vi "String To Anything.vi"(5 "Use Supplied":bool, 7 "Format String (%#_13g)":string="%#_13g", 8 "Error In":errorcluster, 9 "Strings":string[](array[string]), 10 "Type of Anything":variant, 11 "Read/Write Options":T1) -> (0 "Error Out":errorcluster, 3 "Variant":variant)   [LabVIEW 2020]
uses:
  SubVIs/Read Write Options Cluster.ctl
  SubVIs/Read Write Tag Lookup Cluster.ctl
  <vilib>/Utility/VariantDataType/Type.ctl
  <vilib>/Utility/VariantDataType/VariantType.lvlib
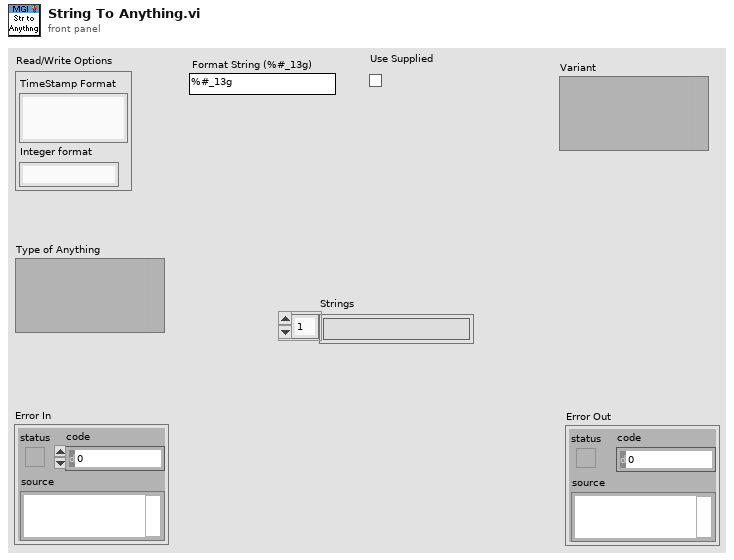
[diagram p1: front panel]
types:
  T1 = typedef "Read Write Options Cluster.ctl" = cluster{"TimeStamp Format":string, "Integer format":string}
  T2 = typedef "Read Write Tag Lookup Cluster.ctl" = cluster{"StrToSpecifiedText":variant, "Specified Data":variant, "Options":T1, "FloatFormat":string}
  T3 = typedef "VariantType.lvlib/Type.ctl" = enum8{"Invalid Type", "Void", "I8", "I16", "I32", "I64", "U8", "U16", "U32", "U64", "Single Float", "Double Float", "Extended Float", "Single Complex", "Double Complex", "Extended Complex", "Enum U8", "Enum U16", "Enum U32", "Enum U64", "Single Float With Unit", "Double Float With Unit", "Extended Float With Unit", "Single Complex with Unit", "Double Complex with Unit", "Extended Complex with Unit", "Boolean", "String", "Path", "Picture", "Tag", "Array", "Cluster", "Variant", "LV Variant", "Waveform", "Timestamp", "Digital Waveform", "Digital Data", "ExpressData", "Refnum", "External Data", "VI", "Poly VI", "LabVIEW Class Instance", "Fixed Point"}
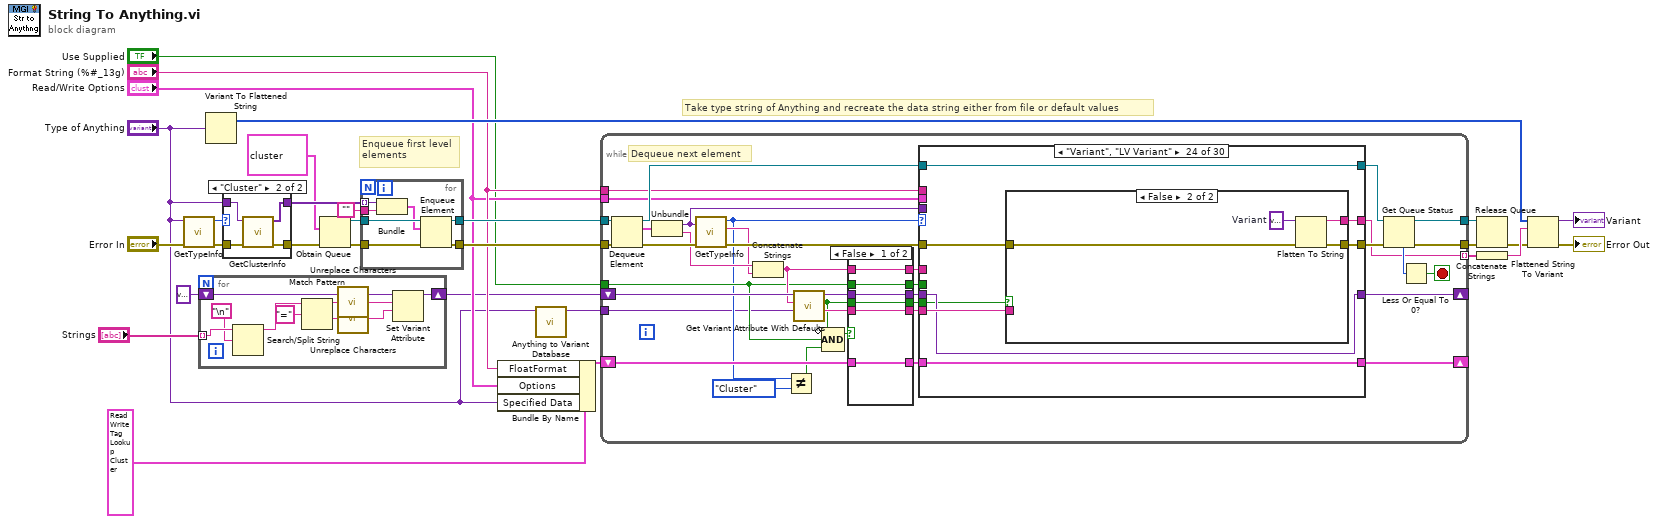
[diagram p0: block diagram]
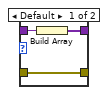
[diagram p2: hidden frame]
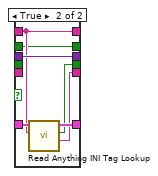
[diagram p3: hidden frame]
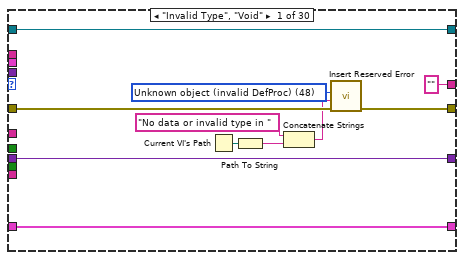
[diagram p4: hidden frame]
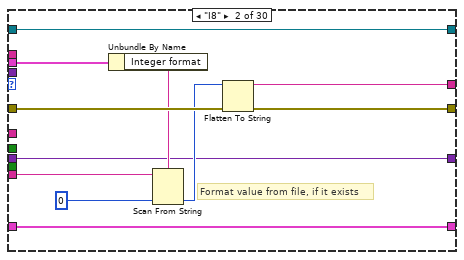
[diagram p5: hidden frame]
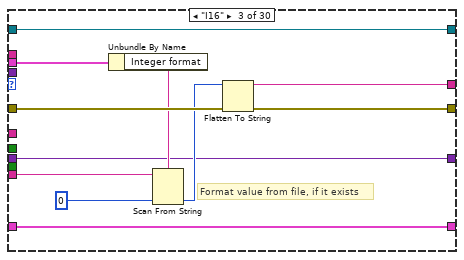
[diagram p6: hidden frame]
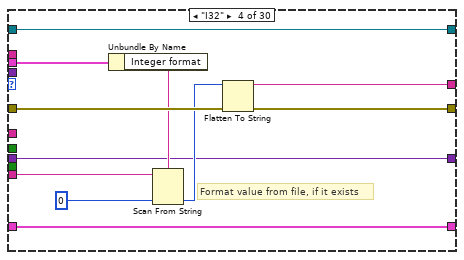
[diagram p7: hidden frame]
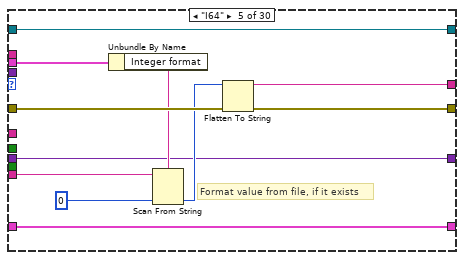
[diagram p8: hidden frame]
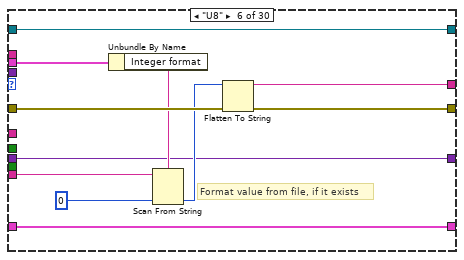
[diagram p9: hidden frame]
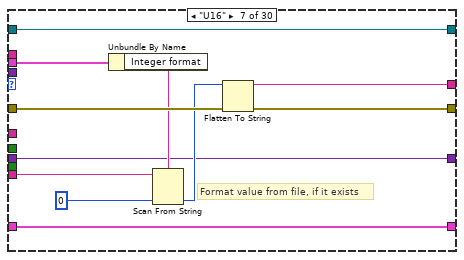
[diagram p10: hidden frame]
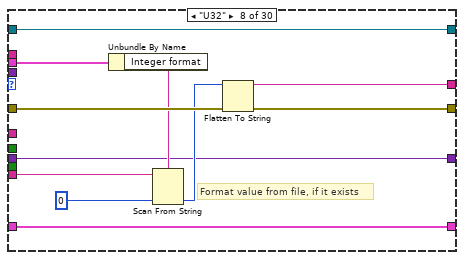
[diagram p11: hidden frame]
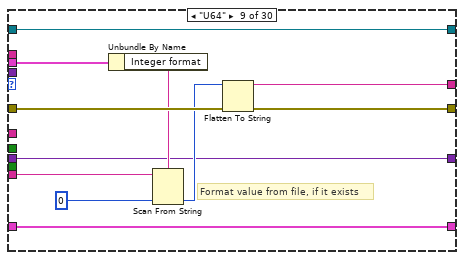
[diagram p12: hidden frame]
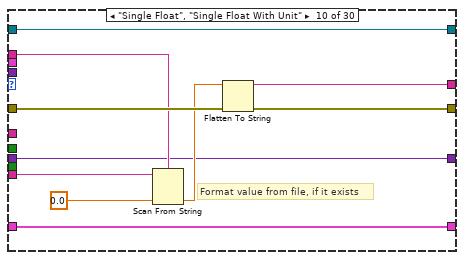
[diagram p13: hidden frame]
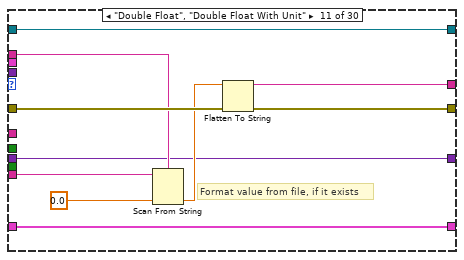
[diagram p14: hidden frame]
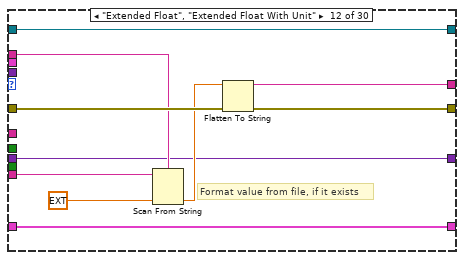
[diagram p15: hidden frame]
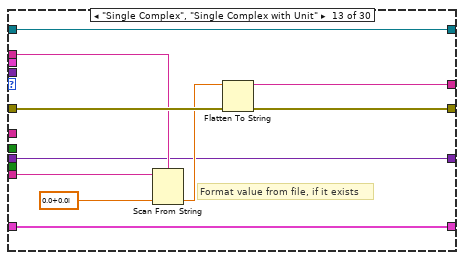
[diagram p16: hidden frame]
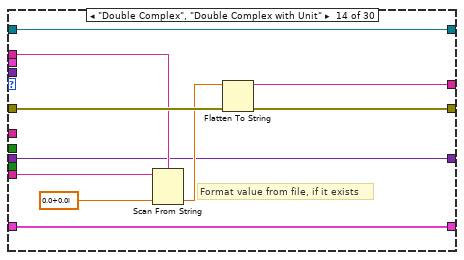
[diagram p17: hidden frame]
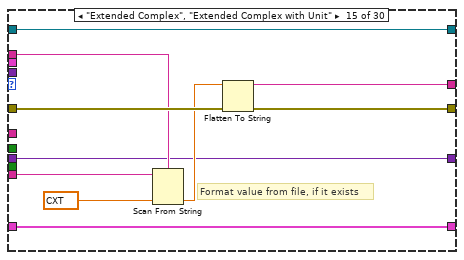
[diagram p18: hidden frame]
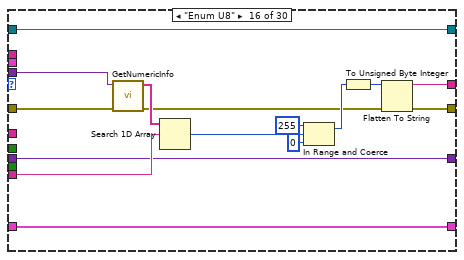
[diagram p19: hidden frame]
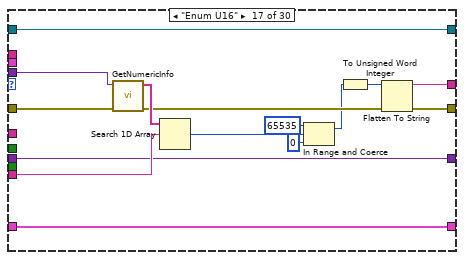
[diagram p20: hidden frame]
diagram:
  # "Enqueue first level\nelements"
  # "Take type string of Anything and recreate the data string either from file or default values"
  n1 = call <vilib>:"GetTypeInfo.vi"("error in (no error)"="Error In", "Variant"="Type of Anything") -> ("error out"=w27:errorcluster, "Type Enum"=w25:T3)  [unwired: 5 in, 3 out]
  n2 = for {
    shift-right: [w37] -> w5
    shift-left: variant ("variant") -> [w38]
    tunnel: "Strings" -> [w32] mode=indexing
    n3 = Search/Split String(string=w32, search string/char (-)="\n") -> (substring before match=w30:string)  [unwired: 1 in, 2 out]
    n4 = Match Pattern(string=w30, regular expression="=") -> (before substring=w36:string, after substring=w35:string)  [unwired: 1 in, 2 out]
    n5 = call "Unreplace Characters.vi"("String In"=w36) -> ("String Out"=w34:string)  [unwired: 1 in]
    n6 = call "Unreplace Characters.vi"("String In"=w35) -> ("String Out"=w33:string)  [unwired: 1 in]
    n7 = Set Variant Attribute(Variant=w38, name=w34, value=w33) -> (Variant out=w37:variant)  [unwired: 1 in, 2 out]
  }
  n8 = Variant To Flattened String(Variant="Type of Anything") -> (1:w10:i16[])  [unwired: 1 out]
  n9 = case shown="\"Cluster\"" w25 {
    tunnel: [w42 w45] -> w26
    tunnel: w27 -> [w42 w46]
    tunnel: "Type of Anything" -> [w41 w44]
    tunnel: [w40 w43] -> w28
    frame Default {
      n10 = Build Array(w41) -> (w40:variant[])
    }
    frame "Cluster" {
      n11 = call <vilib>:"GetClusterInfo.vi"("error in (no error)"=w46, "Variant"=w44) -> ("error out"=w45:errorcluster, "Cluster Elements"=w43:variant[])  [unwired: 8 in]
    }
  }
  n12 = Obtain Queue(element data type=cluster{"Variant":variant, "Name":string} {"Variant"=variant, "Name"=""}, error in (no error)=w26) -> (queue out=w14:refnum<queue>, error out=w22:errorcluster)  [unwired: 3 in, 1 out]
  n13 = for {
    tunnel: w14 -> [w53]
    tunnel: [w52] -> w15
    tunnel: [w51] -> w16
    tunnel: w28 -> [w50] mode=indexing
    tunnel: "" -> [w48]
    tunnel: w22 -> [w47]
    n14 = Bundle("ArrayElt"=w50, w48) -> (w49:cluster{"ArrayElt":variant, string})  [unwired: 1 in]
    n15 = Enqueue Element(queue=w53, element=w49, error in (no error)=w47) -> (queue out=w51:refnum<queue>, error out=w52:errorcluster)  [unwired: 1 in, 1 out]
  }
  n16 = Bundle By Name(cluster=T2 {"StrToSpecifiedText"=variant, "Specified Data"=variant, "Options"={"TimeStamp Format"="", "Integer format"=""}, "FloatFormat"=""} ("State In"), "FloatFormat"="Format String (%#_13g)", "Options"="Read/Write Options", "Specified Data"="Type of Anything") -> (w8:T2)
  n17 = call "Anything to Variant Database.vi"("Type of Anything"="Type of Anything") -> ("Variant Database"=w1:variant)  [unwired: 9 in, 1 out]
  n18 = while {
    tunnel: w15 -> [w90]
    tunnel: [w85] -> w17
    tunnel: [w76] -> w13 mode=indexing
    tunnel: w16 -> [w87]
    tunnel: [w81] -> w19
    tunnel: "Read/Write Options" -> [w75]
    tunnel: "Format String (%#_13g)" -> [w74]
    shift-right: [w59] -> _
    shift-left: w8 -> [w63]
    shift-right: [w58] -> _
    shift-left: w5 -> [w73]
    tunnel: "Use Supplied" -> [w62]
    tunnel: w1 -> [w54]
    stop <- w82 stop-if-true
    # "Dequeue next element"
    n19 = Dequeue Element(queue=w87, error in (no error)=w90) -> (queue out=w88:refnum<queue>, element=w80:cluster{"Variant":variant, "Name":string}, error out=w89:errorcluster)  [unwired: 1 in, 1 out]
    n20 = Unbundle(w80) -> ("Variant"=w78:variant, "Name"=w79:string)
    n21 = call <vilib>:"GetTypeInfo.vi"("error in (no error)"=w89, "Variant"=w78) -> ("error out"=w91:errorcluster, "Name"=w77:string, "Type Enum"=w57:T3)  [unwired: 5 in, 2 out]
    n22 = Concatenate Strings(w79, w77) -> (w69:string)
    n23 = Not Equal?(x=w57, y=Type."Cluster") -> (x != y?=w56:bool)
    n24 = call "Get Variant Attribute With Defaults.vi"("Variant Database defaults"=w54, "name"=w69, "Variant Database from file"=w73) -> ("values"=w72:string, "found"=w71:bool, "Variant out"=w68:variant)  [unwired: 6 in]
    n25 = Compound Arithmetic op=AND(invert w71, w62, w56) -> (w70:bool)
    n26 = case shown="False" w70 {
      tunnel: w72 -> [w94 _]
      tunnel: w71 -> [w95 _]
      tunnel: w69 -> [w96 w99]
      tunnel: w68 -> [w97 w103]
      tunnel: [w97 w103] -> w67
      tunnel: [w96 w99] -> w66
      tunnel: [w95 w101] -> w65
      tunnel: [w94 w100] -> w64
      tunnel: w63 -> [w93 w104]
      tunnel: [w93 w102] -> w60
      tunnel: w62 -> [w92 w98]
      tunnel: [w92 w98] -> w61
      frame False {
      }
      frame True {
        n27 = call "Read Anything INI Tag Lookup.vi"("Str"=w99, "State In"=w104) -> ("INI Text"=w100:string, "Text Found?"=w101:bool, "State Out"=w102:T2)  [unwired: 7 in]
      }
    }
    n28 = case shown="\"Variant\", \"LV Variant\"" w57 {
      tunnel: [w109 w126 w137 w148 w159 w170 w181 w192 w203 w213 w223 w233 w243 w253 w263 w278 w293 w308 w323 w333 w341 w349 w357 w378 w406 w439 w481 w509 w540 w552] -> w86
      tunnel: w91 -> [w110 w125 w136 w147 w158 w169 w180 w191 w202 w212 w222 w232 w242 w252 w262 w277 w292 w307 w322 w332 w340 w348 w363 w377 w405 w438 w480 w508 w543 w551]
      tunnel: w66 -> [_ _ _ _ _ _ _ _ _ _ _ _ _ _ _ _ _ _ _ _ _ _ w350 _ _ _ _ _ w537 _]
      tunnel: ["" ("data string") w124 w135 w146 w157 w168 w179 w190 w201 w211 w221 w231 w241 w251 w261 w276 w291 w306 w321 w331 w339 w347 "" w376 w404 w437 w479 w507 w532 w550] -> w76
      tunnel: w78 -> [_ _ _ _ _ _ _ _ _ _ _ _ _ _ _ w275 w290 w305 w320 _ _ _ w362 _ _ _ _ _ w542 _]
      tunnel: w88 -> [w111 w123 w134 w145 w156 w167 w178 w189 w200 w210 w220 w230 w240 w250 w260 w274 w289 w304 w319 w330 w338 w346 w358 w375 w403 w436 w478 w506 w544 w549]
      tunnel: [w111 w123 w134 w145 w156 w167 w178 w189 w200 w210 w220 w230 w240 w250 w260 w274 w289 w304 w319 w330 w338 w346 w356 w375 w403 w436 w478 w506 w539 w549] -> w84
      tunnel: w67 -> [w106 w117 w128 w139 w150 w161 w172 w183 w195 w205 w215 w225 w235 w246 w255 w265 w280 w295 w310 w325 w336 w343 w352 w373 w400 w428 w475 w503 w536 w546]
      tunnel: w75 -> [_ w122 w133 w144 w155 w166 w177 w188 w199 _ _ _ _ _ _ _ _ _ _ _ _ _ _ _ _ w435 _ _ w531 _]
      tunnel: w74 -> [_ _ _ _ _ _ _ _ _ w207 w217 w227 w237 w247 w257 _ _ _ _ _ _ _ _ _ _ _ _ _ w530 _]
      tunnel: [w106 w117 w128 w139 w150 w161 w172 w183 w195 w205 w215 w225 w235 w246 w255 w265 w280 w295 w310 w325 w336 w343 w352 w373 w400 w428 w475 w503 w533 w546] -> w58
      tunnel: w64 -> [_ w118 w129 w140 w151 w162 w173 w184 w194 w206 w216 w226 w236 w245 w256 w266 w281 w296 w311 w326 w337 w344 _ w374 w402 w429 w476 w504 w541 w547]
      tunnel: w65 -> [_ _ _ _ _ _ _ _ _ _ _ _ _ _ _ _ _ _ _ _ _ _ _ w372 w401 w430 w477 w505 _ w548]
      tunnel: w61 -> [_ _ _ _ _ _ _ _ _ _ _ _ _ _ _ _ _ _ _ _ _ _ _ _ _ _ _ _ w538 _]
      tunnel: w60 -> [w105 w116 w127 w138 w149 w160 w171 w182 w193 w204 w214 w224 w234 w244 w254 w264 w279 w294 w309 w324 w335 w342 w351 w371 w399 w427 w474 w502 w535 w545]
      tunnel: [w105 w116 w127 w138 w149 w160 w171 w182 w193 w204 w214 w224 w234 w244 w254 w264 w279 w294 w309 w324 w335 w342 w351 w371 w399 w427 w474 w502 w534 w545] -> w59
      frame "Invalid Type", "Void" {
        w107 = u16 48 items=["No error", "Argument error", "Memory is full", "Out of zone", "End of file", "File already open", "Generic file I/O error", "File not found", "File permission error", "Disk is full", "Duplicate path", "Too many files open", "System feature not enabled", "Resource file not found", "Cannot add resource", "Resource not found", "Image not found", "Image memory error", "Pen does not exist", "Config type invalid", "Config token not found", "Config parse error", "Config memory error", "Bad external code format", "Bad external code offset", "External code not present", "Null window", "Destroy window error", "Null menu", "Print aborted", "Bad print record", "Print driver error", "Windows error during printing", "Memory error during printing", "Print dialog error", "Generic print error", "Invalid device refnum", "Device not found", "Device parameter error", "Device unit error", "Cannot open device", "Device call aborted", "Generic error", "Cancelled by user", "Object ID too low", "Object ID too high", "Object not in heap", "Unknown heap", "Unknown object (invalid DefProc)", "Unknown object (DefProc not in table)", "Message out of range", "Invalid (null) method", "Unknown message", "Manager call not supported", "Bad address", "Network operation in progress", "Network operation timed out", "Connection is busy", "Network attribute not supported", "Network error", "Address in use", "System out of memory", "Connection aborted", "Connection refused", "Not connected", "Already connected", "Connection closed", "Initialization error (interapplication manager)", "Bad occurrence", "Wait on unbound occurrence handler", "Occurrence queue overflow", "Datalog type conflict", "Unused", "Unrecognized type (interapplication manager)", "Memory corrupt", "Failed to make temporary DLL", "Old CIN version", "Drag socket not found", "Failed to load drop-object", "Failed to register OLE object", "Failed to release OLE object", "Format specifier type mismatch", "Unknown format specifier", "Too few format specifiers", "Too many format specifiers", "Scan failed", "Newer CIN version", "OLE Convert", "Runtime menu error", "Password tampered", "Unknown error code"] ("Reserved Error Code")
        n29 = Current VI's Path() -> (path=w113:path)
        n30 = Path To String(path=w113) -> (string=w112:string)
        n31 = Concatenate Strings("No data or invalid type in " ("string"), w112) -> (w108:string)
        n32 = call "Insert Reserved Error.vi"("error in (no error)"=w110, "non-standard source (\"\")"=w108, "Reserved Error Code"=w107) -> ("error out"=w109:errorcluster)  [unwired: 4 in]
      }
      frame "I8" {
        # "Format value from file, if it exists"
        n33 = Unbundle By Name(w122) -> ("Integer format"=w120:string)
        n34 = Scan From String(format string=w120, input string=w118, default 1=i8 0 ("default (0 I32)")) -> (output 1=w119:i8)  [unwired: 2 in, 3 out]
        n35 = Flatten To String(anything=w119, error in (no error)=w125) -> (data string=w124:string, error out=w126:errorcluster)  [unwired: 2 in, 1 out]
      }
      frame "I16" {
        # "Format value from file, if it exists"
        n36 = Unbundle By Name(w133) -> ("Integer format"=w131:string)
        n37 = Scan From String(format string=w131, input string=w129, default 1=i16 0 ("default (0 I32)")) -> (output 1=w130:i16)  [unwired: 2 in, 3 out]
        n38 = Flatten To String(anything=w130, error in (no error)=w136) -> (data string=w135:string, error out=w137:errorcluster)  [unwired: 2 in, 1 out]
      }
      frame "I32" {
        # "Format value from file, if it exists"
        n39 = Unbundle By Name(w144) -> ("Integer format"=w142:string)
        n40 = Scan From String(format string=w142, input string=w140, default 1=0 ("default (0 I32)")) -> (output 1=w141:i32)  [unwired: 2 in, 3 out]
        n41 = Flatten To String(anything=w141, error in (no error)=w147) -> (data string=w146:string, error out=w148:errorcluster)  [unwired: 2 in, 1 out]
      }
      frame "I64" {
        # "Format value from file, if it exists"
        n42 = Unbundle By Name(w155) -> ("Integer format"=w153:string)
        n43 = Scan From String(format string=w153, input string=w151, default 1=i64 0 ("default (0 I32)")) -> (output 1=w152:i64)  [unwired: 2 in, 3 out]
        n44 = Flatten To String(anything=w152, error in (no error)=w158) -> (data string=w157:string, error out=w159:errorcluster)  [unwired: 2 in, 1 out]
      }
      frame "U8" {
        # "Format value from file, if it exists"
        n45 = Unbundle By Name(w166) -> ("Integer format"=w164:string)
        n46 = Scan From String(format string=w164, input string=w162, default 1=u8 0 ("default (0 I32)")) -> (output 1=w163:u8)  [unwired: 2 in, 3 out]
        n47 = Flatten To String(anything=w163, error in (no error)=w169) -> (data string=w168:string, error out=w170:errorcluster)  [unwired: 2 in, 1 out]
      }
      frame "U16" {
        # "Format value from file, if it exists"
        n48 = Unbundle By Name(w177) -> ("Integer format"=w175:string)
        n49 = Scan From String(format string=w175, input string=w173, default 1=u16 0 ("default (0 I32)")) -> (output 1=w174:u16)  [unwired: 2 in, 3 out]
        n50 = Flatten To String(anything=w174, error in (no error)=w180) -> (data string=w179:string, error out=w181:errorcluster)  [unwired: 2 in, 1 out]
      }
      frame "U32" {
        # "Format value from file, if it exists"
        n51 = Unbundle By Name(w188) -> ("Integer format"=w186:string)
        n52 = Scan From String(format string=w186, input string=w184, default 1=u32 0 ("default (0 I32)")) -> (output 1=w185:u32)  [unwired: 2 in, 3 out]
        n53 = Flatten To String(anything=w185, error in (no error)=w191) -> (data string=w190:string, error out=w192:errorcluster)  [unwired: 2 in, 1 out]
      }
      frame "U64" {
        # "Format value from file, if it exists"
        n54 = Unbundle By Name(w199) -> ("Integer format"=w197:string)
        n55 = Scan From String(format string=w197, input string=w194, default 1=u64 0 ("default (0 I32)")) -> (output 1=w196:u64)  [unwired: 2 in, 3 out]
        n56 = Flatten To String(anything=w196, error in (no error)=w202) -> (data string=w201:string, error out=w203:errorcluster)  [unwired: 2 in, 1 out]
      }
      frame "Single Float", "Single Float With Unit" {
        # "Format value from file, if it exists"
        n57 = Scan From String(format string=w207, input string=w206, default 1=sgl 0.0 ("default (0 I32)")) -> (output 1=w208:sgl)  [unwired: 2 in, 3 out]
        n58 = Flatten To String(anything=w208, error in (no error)=w212) -> (data string=w211:string, error out=w213:errorcluster)  [unwired: 2 in, 1 out]
      }
      frame "Double Float", "Double Float With Unit" {
        # "Format value from file, if it exists"
        n59 = Scan From String(format string=w217, input string=w216, default 1=0.0 ("default (0 I32)")) -> (output 1=w218:dbl)  [unwired: 2 in, 3 out]
        n60 = Flatten To String(anything=w218, error in (no error)=w222) -> (data string=w221:string, error out=w223:errorcluster)  [unwired: 2 in, 1 out]
      }
      frame "Extended Float", "Extended Float With Unit" {
        # "Format value from file, if it exists"
        n61 = Scan From String(format string=w227, input string=w226, default 1=ext 0.0 ("default (0 I32)")) -> (output 1=w228:ext)  [unwired: 2 in, 3 out]
        n62 = Flatten To String(anything=w228, error in (no error)=w232) -> (data string=w231:string, error out=w233:errorcluster)  [unwired: 2 in, 1 out]
      }
      frame "Single Complex", "Single Complex with Unit" {
        # "Format value from file, if it exists"
        n63 = Scan From String(format string=w237, input string=w236, default 1=csg 0.0+0.0i ("default (0 I32)")) -> (output 1=w238:csg)  [unwired: 2 in, 3 out]
        n64 = Flatten To String(anything=w238, error in (no error)=w242) -> (data string=w241:string, error out=w243:errorcluster)  [unwired: 2 in, 1 out]
      }
      frame "Double Complex", "Double Complex with Unit" {
        # "Format value from file, if it exists"
        n65 = Scan From String(format string=w247, input string=w245, default 1=cdb 0.0+0.0i ("default (0 I32)")) -> (output 1=w248:cdb)  [unwired: 2 in, 3 out]
        n66 = Flatten To String(anything=w248, error in (no error)=w252) -> (data string=w251:string, error out=w253:errorcluster)  [unwired: 2 in, 1 out]
      }
      frame "Extended Complex", "Extended Complex with Unit" {
        # "Format value from file, if it exists"
        n67 = Scan From String(format string=w257, input string=w256, default 1=cxt 0.0+0.0i ("default (0 I32)")) -> (output 1=w258:cxt)  [unwired: 2 in, 3 out]
        n68 = Flatten To String(anything=w258, error in (no error)=w262) -> (data string=w261:string, error out=w263:errorcluster)  [unwired: 2 in, 1 out]
      }
      frame "Enum U8" {
        n69 = call <vilib>:"GetNumericInfo.vi"("error in (no error)"=w277, "Variant"=w275) -> ("error out"=w267:errorcluster, "EnumNames"=w273:string[])  [unwired: 6 in, 2 out]
        n70 = Search 1D Array(1D array=w273, element=w266) -> (index of element=w272:i32)  [unwired: 1 in]
        n71 = In Range and Coerce(upper limit=255, x=w272, lower limit=0) -> (coerced(x)=w270:i32)  [unwired: 1 out]
        n72 = To Unsigned Byte Integer(number=w270) -> (unsigned 8bit integer=w271:u8)
        n73 = Flatten To String(anything=w271, error in (no error)=w267) -> (data string=w276:string, error out=w278:errorcluster)  [unwired: 2 in, 1 out]
      }
      frame "Enum U16" {
        n74 = call <vilib>:"GetNumericInfo.vi"("error in (no error)"=w292, "Variant"=w290) -> ("error out"=w285:errorcluster, "EnumNames"=w288:string[])  [unwired: 6 in, 2 out]
        n75 = Search 1D Array(1D array=w288, element=w281) -> (index of element=w287:i32)  [unwired: 1 in]
        n76 = In Range and Coerce(upper limit=u16 65535, x=w287, lower limit=0) -> (coerced(x)=w283:i32)  [unwired: 1 out]
        n77 = To Unsigned Word Integer(number=w283) -> (unsigned 16bit integer=w282:u16)
        n78 = Flatten To String(anything=w282, error in (no error)=w285) -> (data string=w291:string, error out=w293:errorcluster)  [unwired: 2 in, 1 out]
      }
      frame "Enum U32" {
        n79 = call <vilib>:"GetNumericInfo.vi"("error in (no error)"=w307, "Variant"=w305) -> ("error out"=w300:errorcluster, "EnumNames"=w303:string[])  [unwired: 6 in, 2 out]
        n80 = Search 1D Array(1D array=w303, element=w296) -> (index of element=w302:i32)  [unwired: 1 in]
        n81 = In Range and Coerce(upper limit=u32 4294967295, x=w302, lower limit=u32 0) -> (coerced(x)=w299:u32)  [unwired: 1 out]
        n82 = To Unsigned Long Integer(number=w299) -> (unsigned 32bit integer=w298:u32)
        n83 = Flatten To String(anything=w298, error in (no error)=w300) -> (data string=w306:string, error out=w308:errorcluster)  [unwired: 2 in, 1 out]
      }
      frame "Enum U64" {
        n84 = call <vilib>:"GetNumericInfo.vi"("error in (no error)"=w322, "Variant"=w320) -> ("error out"=w315:errorcluster, "EnumNames"=w318:string[])  [unwired: 6 in, 2 out]
        n85 = Search 1D Array(1D array=w318, element=w311) -> (index of element=w317:i32)  [unwired: 1 in]
        n86 = In Range and Coerce(upper limit=2147483647, x=w317, lower limit=0) -> (coerced(x)=w312:i32)  [unwired: 1 out]
        n87 = To Unsigned Quad Integer(1:w312) -> (0:w313:u64)
        n88 = Flatten To String(anything=w313, error in (no error)=w315) -> (data string=w321:string, error out=w323:errorcluster)  [unwired: 2 in, 1 out]
      }
      frame "Boolean" {
        n89 = call <vilib>:"Trim Whitespace.vi"("string"=w326) -> ("trimmed string"=w328:string)  [unwired: 1 in]
        n90 = To Upper Case(1:w328) -> (0:w327:string)
        n91 = case shown="Default" w327 {
          tunnel: [_ TRUE] -> w329
          frame Default {
          }
          frame "1", "ON", "TRUE", "YES" {
          }
        }
        n92 = Flatten To String(anything=w329, error in (no error)=w332) -> (data string=w331:string, error out=w333:errorcluster)  [unwired: 2 in, 1 out]
      }
      frame "String" {
        n93 = Flatten To String(anything=w337, error in (no error)=w340) -> (data string=w339:string, error out=w341:errorcluster)  [unwired: 2 in, 1 out]
      }
      frame "Path" {
        n94 = String To Path(string=w344) -> (path=w345:path)
        n95 = Flatten To String(anything=w345, error in (no error)=w348) -> (data string=w347:string, error out=w349:errorcluster)  [unwired: 2 in, 1 out]
      }
      frame "Cluster" {
        # "Enqueue cluster elements"
        n96 = call <vilib>:"GetClusterInfo.vi"("error in (no error)"=w363, "Variant"=w362) -> ("error out"=w359:errorcluster, "Cluster Elements"=w361:variant[])  [unwired: 8 in]
        n97 = Concatenate Strings(w350, "." ("string")) -> (w353:string)
        n98 = Reverse 1D Array(array=w361) -> (reversed array=w360:variant[])
        n99 = for {
          tunnel: w358 -> [w370]
          tunnel: w359 -> [w369]
          tunnel: [w368] -> w357
          tunnel: [w367] -> w356
          tunnel: w360 -> [w366] mode=indexing
          tunnel: w353 -> [w364]
          n100 = Bundle("ArrayElt"=w366, w364) -> (w365:cluster{"ArrayElt":variant, string})  [unwired: 1 in]
          n101 = Enqueue Element At Opposite End(queue=w370, element=w365, error in (no error)=w369) -> (queue out=w367:refnum<queue>, error out=w368:errorcluster)  [unwired: 1 in, 1 out]
        }
      }
      frame "Variant", "LV Variant" {
        n102 = case shown="False" w372 {
          tunnel: w374 -> [w379 _]
          tunnel: [w387 w396] -> w378
          tunnel: w377 -> [w387 w397]
          tunnel: [w385 w398] -> w376
          frame True {
            n103 = String Subset(string=w379, offset (0)=2) -> (substring=w384:string)  [unwired: 1 in]
            n104 = String Length(string=w384) -> (length=w382:i32)
            n105 = Multiply(x=0.5, y=w382) -> (x*y=w381:dbl)
            n106 = for {
              N: w381 -> [_]
              tunnel: w384 -> [w391]
              tunnel: [w393] -> w383 mode=indexing
              i -> [w390]
              w389 = 2 ("length (rest)")
              n107 = Multiply(x=w390, y=w389) -> (x*y=w388:i32)
              n108 = String Subset(string=w391, offset (0)=w388, length (rest)=w389) -> (substring=w392:string)
              n109 = Hexadecimal String To Number(string=w392, default (0uL)=u8 0 ("default (0 U32)")) -> (number=w393:u8)  [unwired: 1 in, 1 out]
            }
            n110 = Byte Array To String(unsigned byte array=w383) -> (string=w385:string)
          }
          frame False {
            w395 = variant  # Variant
            n111 = Flatten To String(anything=w395, error in (no error)=w397) -> (data string=w398:string, error out=w396:errorcluster)  [unwired: 2 in, 1 out]
          }
        }
      }
      frame "Waveform" {
        n112 = case shown="True" w401 {
          tunnel: w402 -> [w407 _]
          tunnel: [w415 w425] -> w406
          tunnel: w405 -> [w415 w424]
          tunnel: [w413 w426] -> w404
          frame True {
            n113 = String Subset(string=w407, offset (0)=2) -> (substring=w412:string)  [unwired: 1 in]
            n114 = String Length(string=w412) -> (length=w410:i32)
            n115 = Multiply(x=0.5, y=w410) -> (x*y=w409:dbl)
            n116 = for {
              N: w409 -> [_]
              tunnel: w412 -> [w419]
              tunnel: [w421] -> w411 mode=indexing
              i -> [w418]
              w417 = 2 ("length (rest)")
              n117 = Multiply(x=w418, y=w417) -> (x*y=w416:i32)
              n118 = String Subset(string=w419, offset (0)=w416, length (rest)=w417) -> (substring=w420:string)
              n119 = Hexadecimal String To Number(string=w420, default (0uL)=u8 0 ("default (0 U32)")) -> (number=w421:u8)  [unwired: 1 in, 1 out]
            }
            n120 = Byte Array To String(unsigned byte array=w411) -> (string=w413:string)
          }
          frame False {
            n121 = Flatten To String(anything=waveform(dbl) {"t0"=timestamp(0 s since 1904-01-01), "dt"=0.0, "Y"=[]} ("Waveform 2"), error in (no error)=w424) -> (data string=w426:string, error out=w425:errorcluster)  [unwired: 2 in, 1 out]
          }
        }
      }
      frame "Timestamp" {
        n122 = Unbundle By Name(w435) -> ("TimeStamp Format"=w434:string)
        n123 = Match First String(2:string[] ["0x"] ("string array"), 3:w429) -> (0:w432:i32, 1:w431:string)
        n124 = case shown="True" w430 {
          tunnel: [w441 w472] -> w439
          tunnel: w438 -> [w442 w471]
          tunnel: [w445 w473] -> w437
          tunnel: w434 -> [w444 _]
          tunnel: w432 -> [w440 _]
          tunnel: w431 -> [w443 _]
          frame True {
            n125 = case shown="0.." w440 {
              tunnel: [w447 w467] -> w445
              tunnel: w444 -> [_ w463]
              tunnel: w443 -> [w449 w466]
              tunnel: w442 -> [w448 w465]
              tunnel: [w448 w464] -> w441
              frame 0.. {
                n126 = String Length(string=w449) -> (length=w450:i32)
                n127 = Quotient & Remainder(x=w450, y=2) -> (floor(x/y)=w452:i32)  [unwired: 1 out]
                n128 = for {
                  N: w452 -> [_]
                  tunnel: w449 -> [w456]
                  tunnel: [w458] -> w446 mode=indexing
                  i -> [w455]
                  w454 = 2 ("length (rest)")
                  n129 = Multiply(x=w455, y=w454) -> (x*y=w453:i32)
                  n130 = String Subset(string=w456, offset (0)=w453, length (rest)=w454) -> (substring=w457:string)
                  n131 = Hexadecimal String To Number(string=w457, default (0uL)=u8 0 ("default (0 U32)")) -> (number=w458:u8)  [unwired: 1 in, 1 out]
                }
                n132 = Byte Array To String(unsigned byte array=w446) -> (string=w447:string)
              }
              frame ..-1 {
                n133 = Concatenate Strings("%<" ("string"), w463, ">T" ("string")) -> (w462:string)
                n134 = Scan From String(format string=w462, input string=w466, default 1=timestamp(0 s since 1904-01-01)) -> (output 1=w468:timestamp)  [unwired: 2 in, 3 out]
                n135 = Flatten To String(anything=w468, error in (no error)=w465) -> (data string=w467:string, error out=w464:errorcluster)  [unwired: 2 in, 1 out]
              }
            }
          }
          frame False {
            n136 = Flatten To String(anything=timestamp(0 s since 1904-01-01), error in (no error)=w471) -> (data string=w473:string, error out=w472:errorcluster)  [unwired: 2 in, 1 out]
          }
        }
      }
      frame "Digital Waveform" {
        n137 = case shown="True" w477 {
          tunnel: w476 -> [w482 _]
          tunnel: [w490 w500] -> w481
          tunnel: w480 -> [w490 w499]
          tunnel: [w488 w501] -> w479
          frame True {
            n138 = String Subset(string=w482, offset (0)=2) -> (substring=w487:string)  [unwired: 1 in]
            n139 = String Length(string=w487) -> (length=w485:i32)
            n140 = Multiply(x=0.5, y=w485) -> (x*y=w484:dbl)
            n141 = for {
              N: w484 -> [_]
              tunnel: w487 -> [w494]
              tunnel: [w496] -> w486 mode=indexing
              i -> [w493]
              w492 = 2 ("length (rest)")
              n142 = Multiply(x=w493, y=w492) -> (x*y=w491:i32)
              n143 = String Subset(string=w494, offset (0)=w491, length (rest)=w492) -> (substring=w495:string)
              n144 = Hexadecimal String To Number(string=w495, default (0uL)=u8 0 ("default (0 U32)")) -> (number=w496:u8)  [unwired: 1 in, 1 out]
            }
            n145 = Byte Array To String(unsigned byte array=w486) -> (string=w488:string)
          }
          frame False {
            n146 = call <vilib>:"DWDT Empty Digital.vi"() -> ("digital waveform out"=w498:digitalwaveform)  [unwired: 5 in]
            n147 = Flatten To String(anything=w498, error in (no error)=w499) -> (data string=w501:string, error out=w500:errorcluster)  [unwired: 2 in, 1 out]
          }
        }
      }
      frame "Digital Data" {
        n148 = case shown="False" w505 {
          tunnel: w504 -> [w510 _]
          tunnel: [w518 w528] -> w509
          tunnel: w508 -> [w518 w527]
          tunnel: [w516 w529] -> w507
          frame True {
            n149 = String Subset(string=w510, offset (0)=2) -> (substring=w515:string)  [unwired: 1 in]
            n150 = String Length(string=w515) -> (length=w513:i32)
            n151 = Multiply(x=0.5, y=w513) -> (x*y=w512:dbl)
            n152 = for {
              N: w512 -> [_]
              tunnel: w515 -> [w522]
              tunnel: [w524] -> w514 mode=indexing
              i -> [w521]
              w520 = 2 ("length (rest)")
              n153 = Multiply(x=w521, y=w520) -> (x*y=w519:i32)
              n154 = String Subset(string=w522, offset (0)=w519, length (rest)=w520) -> (substring=w523:string)
              n155 = Hexadecimal String To Number(string=w523, default (0uL)=u8 0 ("default (0 U32)")) -> (number=w524:u8)  [unwired: 1 in, 1 out]
            }
            n156 = Byte Array To String(unsigned byte array=w514) -> (string=w516:string)
          }
          frame False {
            n157 = call <vilib>:"DTbl Empty Digital.vi"() -> ("digital data"=w526:digitaldata)  [unwired: 5 in]
            n158 = Flatten To String(anything=w526, error in (no error)=w527) -> (data string=w529:string, error out=w528:errorcluster)  [unwired: 2 in, 1 out]
          }
        }
      }
      frame "Array" {
        n159 = call "Unprocess Array Elements V2.vi"("Queue In"=w544, "Value"=w541, "Read/Write Options"=w531, "Format String (%#_13g)"=w530, "Array Variant"=w542, "Name In"=w537, "Str to INI in"=w536, "Error In"=w543, "Use Specified?"=w538, "State In"=w535) -> ("Queue Out"=w539:refnum<queue>, "Data Out"=w532:string, "Str to INI out"=w533:variant, "State Out"=w534:T2, "Error Out"=w540:errorcluster)  [unwired: 1 in]
      }
      frame Default {
        n160 = case shown="True" w548 {
          tunnel: w547 -> [w553 _]
          tunnel: [w561 w570] -> w552
          tunnel: w551 -> [w561 w571]
          tunnel: [w559 w572] -> w550
          frame True {
            n161 = String Subset(string=w553, offset (0)=2) -> (substring=w558:string)  [unwired: 1 in]
            n162 = String Length(string=w558) -> (length=w556:i32)
            n163 = Multiply(x=0.5, y=w556) -> (x*y=w554:dbl)
            n164 = for {
              N: w554 -> [_]
              tunnel: w558 -> [w565]
              tunnel: [w567] -> w557 mode=indexing
              i -> [w564]
              w563 = 2 ("length (rest)")
              n165 = Multiply(x=w564, y=w563) -> (x*y=w562:i32)
              n166 = String Subset(string=w565, offset (0)=w562, length (rest)=w563) -> (substring=w566:string)
              n167 = Hexadecimal String To Number(string=w566, default (0uL)=u8 0 ("default (0 U32)")) -> (number=w567:u8)  [unwired: 1 in, 1 out]
            }
            n168 = Byte Array To String(unsigned byte array=w557) -> (string=w559:string)
          }
          frame False {
            n169 = Flatten To String(anything="", error in (no error)=w571) -> (data string=w572:string, error out=w570:errorcluster)  [unwired: 2 in, 1 out]
          }
        }
      }
    }
    n170 = Get Queue Status(queue=w84, error in (no error)=w86) -> (queue out=w81:refnum<queue>, error out=w85:errorcluster, # elements in queue=w83:i32)  [unwired: 1 in, 5 out]
    n171 = Less Or Equal To 0?(x=w83) -> (x <= 0?=w82:bool)
  }
  n172 = Release Queue(queue=w19, error in (no error)=w17) -> (error out=w18:errorcluster)  [unwired: 1 in, 2 out]
  n173 = Concatenate Strings(w13) -> (w24:string)
  n174 = Flattened String To Variant(4:w18, 6:w24, 7:w10) -> (0:→"Error Out":errorcluster, 3:→"Variant":variant)
